vi "Startup Path.vi"() -> (0 "Startup.ini":path)   [LabVIEW 2018, in "Core.lvlib"]
uses:
  Core.lvlib
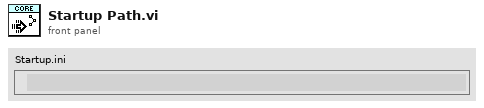
[diagram p1: front panel]
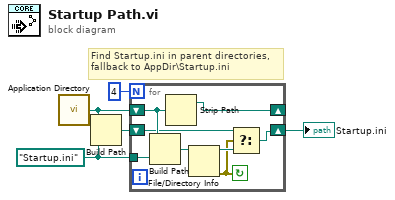
[diagram p0: block diagram]
diagram:
  w3 = path "Startup.ini"
  # "Find Startup.ini in parent directories,\nfallback to AppDir\\Startup.ini"
  n1 = call <vilib>:"Application Directory.vi"() -> ("Application Directory"=w5:path)
  n2 = Build Path(base path=w5, name or relative path=w3) -> (appended path=w4:path)
  n3 = for {
    N: 4 -> [_]
    shift-right: [w7] -> w1
    shift-left: w4 -> [w8]
    shift-right: [w12] -> _
    shift-left: w5 -> [w13]
    tunnel: w3 -> [w11]
    stop <- w6 continue-if-true
    n4 = Build Path(base path=w13, name or relative path=w11) -> (appended path=w10:path)
    n5 = Strip Path(path=w13) -> (stripped path=w12:path)  [unwired: 1 out]
    n6 = File/Directory Info(path=w10) -> (path out=w9:path, error out=w6:errorcluster)  [unwired: 1 in, 5 out]
    n7 = Select(t=w8, s=w6, f=w9) -> (s? t:f=w7:path)
  }
  "Startup.ini" <- w1
